vi "SGUI Set Single Value and Uncertainty to String by Label.vi"(0 "label (empty)":string, 1 "value (empty)":dbl=nan, 2 "uncertainty (empty)":dbl=nan, 3 "unit (empty)":string, 5 "Add SI prefix (true)":bool=TRUE, 7 "error in":errorcluster) -> (4 "control ref out":refnum<vi>, 8 "error out":errorcluster)   [LabVIEW 2013, in "varilib.lvlib"]
doc: "This VI sets '(value ± uncerainty) unit' into string control defined by control label (must be registered first by calling 'SGUI Register Controls'). The formatter also does SI prefix scaling which can be optionally disabled (mostly for unitless quantities). It automatically formats the value and uncertainty to two significant digits of uncertainty. If unit is assigned it will append it after the value and uncertainty. If no value is assigned it will assign empty string (NaN is considered as no input). It will generate error if control not found or has ivalid type but it ignores input errors (executes anyway)."
uses:
  varilib.lvlib
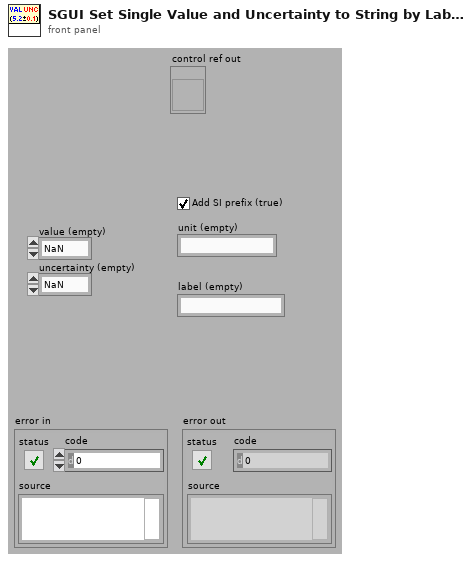
[diagram p1: front panel]
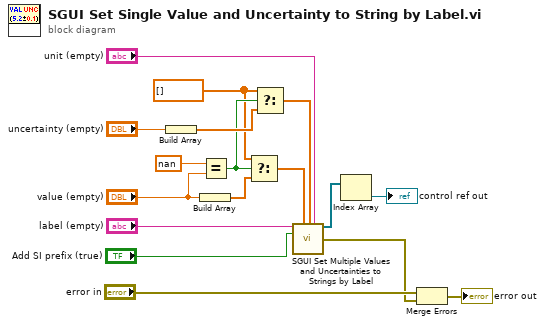
[diagram p0: block diagram]
diagram:
  w7 = dbl[] [] ("t")
  n1 = Build Array("uncertainty (empty)") -> (w10:dbl[])
  n2 = Build Array("value (empty)") -> (w12:dbl[])
  n3 = Equal?(x=nan, y="value (empty)") -> (x = y?=w8:bool)
  n4 = Select(t=w7, s=w8, f=w12) -> (s? t:f=w11:dbl[])
  n5 = Select(t=w7, s=w8, f=w10) -> (s? t:f=w6:dbl[])
  n6 = call "SGUI Set Multiple Values and Uncertainties to Strings by Label.vi"("labels (empty)"="label (empty)", "values (empty)"=w11, "uncertainties (empty)"=w6, "unit (empty)"="unit (empty)", "Add SI prefix (true)"="Add SI prefix (true)") -> ("assigned control refs"=w3:refnum<vi>[], "error out"=w15:errorcluster)  [unwired: 9 in]
  n7 = Index Array(array=w3) -> (element=→"control ref out":refnum<vi>)  [unwired: 1 in]
  n8 = Merge Errors("error in", w15) -> (→"error out":errorcluster)
